vi "PolynomShift.vi"(8 "error in":errorcluster, 9 "CoefficientsBwd":dbl[](array[numeric]) format="%#.4g", 10 "CoefficientsFwd":dbl[](array[numeric]) format="%#.4g") -> (0 "error out":errorcluster, 1 "ShiftedCoefficientsBwd":dbl[](array[numeric]) format="%#.4g", 2 "ShiftedCoefficientsFwd":dbl[](array[numeric]) format="%#.4g")   [LabVIEW 2016]
uses:
  <vilib>/Analysis/Matrix/Numeric/Conversions/Array To Matrix - RA.vi
  <vilib>/Analysis/Matrix/Numeric/Conversions/Array To Matrix - RA2.vi
  <vilib>/Analysis/Matrix/Numeric/Multiply/Multiply - RM,RM.vi
  <vilib>/Analysis/Matrix/Numeric/Conversions/Matrix To Array - RM.vi
  <vilib>/Analysis/Matrix/NI_Matrix.lvlib
panel:
  # "A+Bx+Cxx+Dxxx"
  # "x\" = x - Offset"
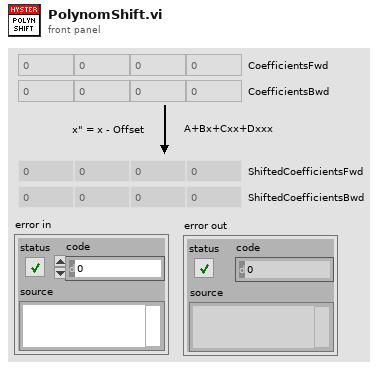
[diagram p1: front panel]
types:
  T1 = typedef "NI_Matrix.lvlib/RealMatrix.ctl" = dbl[][]
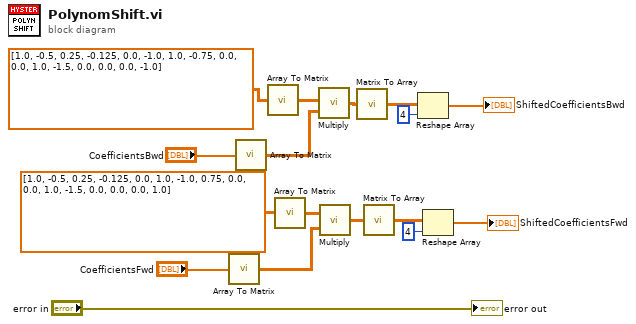
[diagram p0: block diagram]
diagram:
  n1 = call-poly <vilib>:"Array To Matrix.vi"("Real 1D Array"="CoefficientsFwd") -> ("Real Matrix (Column Vector)"=w15:T1)
  n2 = call-poly <vilib>:"Array To Matrix.vi"("Real 1D Array"="CoefficientsBwd") -> ("Real Matrix (Column Vector)"=w7:T1)
  n3 = call-poly <vilib>:"Array To Matrix.vi"("Real 2D Array"=dbl[][] [[1.0, -0.5, 0.25, -0.125], [0.0, -1.0, 1.0, -0.75], [0.0, 0.0, 1.0, -1.5], [0.0, 0.0, 0.0, -1.0]]) -> ("Real Matrix"=w6:T1)
  n4 = call-poly <vilib>:"Array To Matrix.vi"("Real 2D Array"=dbl[][] [[1.0, -0.5, 0.25, -0.125], [0.0, 1.0, -1.0, 0.75], [0.0, 0.0, 1.0, -1.5], [0.0, 0.0, 0.0, 1.0]]) -> ("Real Matrix"=w16:T1)
  n5 = call-poly <vilib>:"Multiply.vi"("Real Matrix B"=w7, "Real Matrix A"=w6) -> ("A * B"=w2:T1)
  n6 = call-poly <vilib>:"Multiply.vi"("Real Matrix B"=w15, "Real Matrix A"=w16) -> ("A * B"=w14:T1)
  n7 = call-poly <vilib>:"Matrix To Array.vi"("Real Matrix"=w2) -> ("Real 2D Array"=w1:dbl[][])
  n8 = call-poly <vilib>:"Matrix To Array.vi"("Real Matrix"=w14) -> ("Real 2D Array"=w13:dbl[][])
  n9 = Reshape Array(w1, 4 ("dimension size")) -> (→"ShiftedCoefficientsBwd":dbl[])
  n10 = Reshape Array(w13, 4 ("dimension size")) -> (→"ShiftedCoefficientsFwd":dbl[])
  "error out" <- "error in"
